vi "json Parse Double Array - array path.vi"(6 "use default?":bool=TRUE, 8 "error in (no error)":errorcluster, 9 "default":dbl[](array[numeric]), 10 "path":string[](array[string]), 11 "JSON Document in":refnum<class "JSON Document.lvclass">) -> (0 "error out":errorcluster, 1 "defaulted?":bool, 2 "value":dbl[](array[numeric]), 3 "JSON Document out":refnum<class "JSON Document.lvclass">, 4 "elements defaulted?":bool[](array[boolean]))   [LabVIEW 2015, in "JSON Document.lvclass"]
uses:
  JSON Document.lvclass
  json Parse Double Array - string path.vi
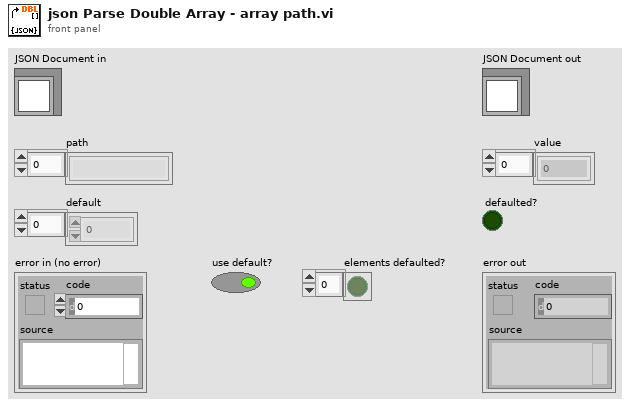
[diagram p1: front panel]
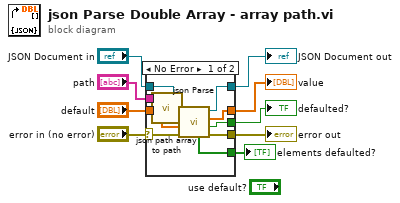
[diagram p0: block diagram]
diagram:
  n1 = case shown="No Error" "error in (no error)" {
    selector: "error in (no error)" -> [w14 w22]
    tunnel: [w13 w22] -> w8
    tunnel: [w18 w21] -> w6
    tunnel: "JSON Document in" -> [w19 w21]
    tunnel: "default" -> [w12 w20]
    tunnel: "path" -> [w15 _]
    tunnel: [w16 w20] -> w3
    tunnel: [w17 _] -> w2
    tunnel: [w11 _] -> w1
    frame No Error {
      n2 = call "json path array to path.vi"("path"=w15) -> ("String"=w10:string)
      n3 = call-poly "json Parse.vi"("error in (no error)"=w14, "default"=w12, "path"=w10, "JSON Document in"=w19) -> ("error out"=w13:errorcluster, "defaulted?"=w17:bool, "value"=w16:dbl[], "JSON Document out"=w18:refnum<class "JSON Document.lvclass">, "elements defaulted?"=w11:bool[])  [unwired: 3 in]
    }
    frame Error {
    }
  }
  "error out" <- w8
  "JSON Document out" <- w6
  "value" <- w3
  "defaulted?" <- w2
  "elements defaulted?" <- w1
